vi "Get Attribute.vi"(5 "Flatten Pointer?":bool, 6 "Include Private?":bool, 7 "Test ID":string, 8 "error in (no error)":errorcluster, 9 "Type":variant, 10 "Attribute Name":string, 11 "Test Executive in":refnum<class "Test Executive.lvclass">) -> (0 "error out":errorcluster, 1 "Attribute":variant, 2 "Attribute Name out":string, 3 "Test Executive out":refnum<class "Test Executive.lvclass">, 4 "Found?":bool)   [LabVIEW 2019, in "Test Executive.lvlib" / "Test Executive.lvclass"]
uses:
  <vilib>/gpm_packages/@cs/test-executive/Source/Test Executive/TestExecutive/Test Executive.lvclass
  <vilib>/gpm_packages/@cs/test-executive/Source/Test Executive/TestExecutive/Test Executive.lvclass/Test Executive.ctl
  2bf17e19-84eb-4e99-8c67-2599d4ea9cd8.vi
  <vilib>/gpm_packages/@cs/linked-list/Source/Linked List/ILinkedList/ILinked List.lvclass
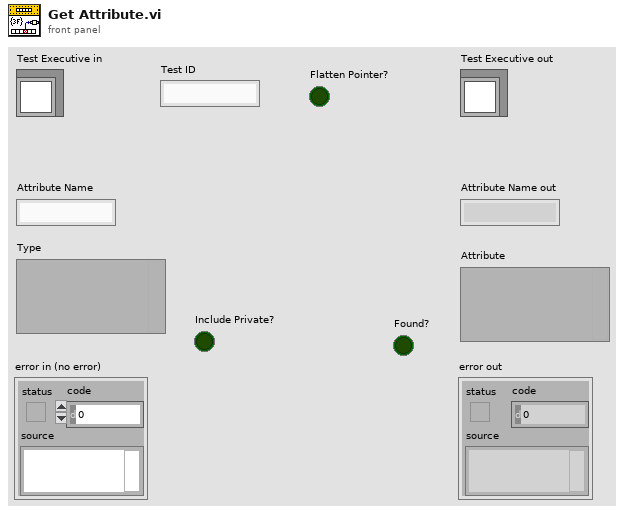
[diagram p1: front panel]
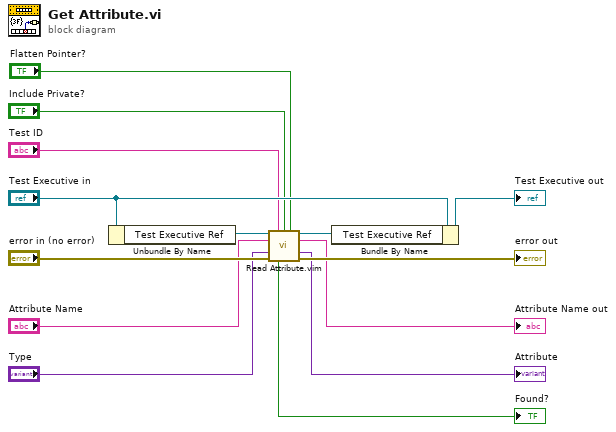
[diagram p0: block diagram]
diagram:
  n1 = Unbundle By Name("Test Executive in") -> ("Test Executive Ref"=w14:refnum<data-value>)
  n2 = call "Read Attribute.vim"("Linked List Ref"=w14, "Linked List ID"="Test ID", "Include Private?"="Include Private?", "Flatten Pointer?"="Flatten Pointer?", "Attribute Name"="Attribute Name", "Type"="Type", "error in (no error)"="error in (no error)") -> ("Linked List Ref out"=w12:refnum<data-value>, "Attribute Name out"=→"Attribute Name out":string, "Attribute"=→"Attribute":variant, "Found?"=→"Found?":bool, "error out"=→"error out":errorcluster)  [unwired: 3 in, 1 out]
  n3 = Bundle By Name(cluster="Test Executive in", "Test Executive Ref"=w12) -> (→"Test Executive out":refnum<class "Test Executive.lvclass">)
